vi "Finish.vi"   [LabVIEW 2019]
doc: "This VIcloses device references, sends final commands to the network tables and the joysticks, and terminates all command and control loops."
uses:
  refnums.vi
  <vilib>/Rock Robotics/WPI/Utilities/WPI_GetSetVariantRefNum.vi
types:
  T1 = typedef "WPI_ServoDeviceRef.ctl" = cluster{"DeviceStatus":errorcluster, "PWM Channel":T2, "DeadBand":T3}
  T2 = typedef "FPGA_DIOPWMChannel.ctl" = enum8{"PWM 0", "PWM 1", "PWM 2", "PWM 3", "PWM 4", "PWM 5", "PWM 6", "PWM 7", "PWM 8", "PWM 9", "PWM MXP 0", "PWM MXP 1", "PWM MXP 2", "PWM MXP 3", "PWM MXP 4", "PWM MXP 5", "PWM MXP 6", "PWM MXP 7", "PWM MXP 8", "PWM MXP 9", "Invalid"}
  T3 = typedef "WPI_PWMDeadband.ctl" = cluster{"Name":string, "maxPositivePwm":i32, "minPositivePwm":i32, "centerPwm":i32, "maxNegativePwm":i32, "minNegativePwm":i32, "angularRange":u16}
  T4 = typedef "WPI_CounterDevRef.ctl" = cluster{"DevStatus":errorcluster, "CntIndex":T5}
  T5 = typedef "FPGA_CounterCtrSystemIndex.ctl" = enum8{"Ctr 0", "Ctr 1", "Ctr 2", "Ctr 3", "Ctr 4", "Ctr 5", "Ctr 6", "Ctr 7", "Invalid"}
  T6 = typedef "WPI_SolenoidDevRef.ctl" = cluster{"DevStatus":errorcluster, "Pneumatics Control Module":u8, "Forward Solenoid Channel":T7, "Reverse Solenoid Channel":T7}
  T7 = typedef "WPI_SolenoidChannel.ctl" = enum8{"Solenoid 0", "Solenoid 1", "Solenoid 2", "Solenoid 3", "Solenoid 4", "Solenoid 5", "Solenoid 6", "Solenoid 7", "Invalid"}
  T8 = typedef "WPI_PotentiometerDevRef.ctl" = cluster{"DevStatus":errorcluster, "Analog Channel":T9, "Invert Output":bool}
  T9 = typedef "FPGA_AIChannel.ctl" = enum8{"AI 0", "AI 1", "AI 2", "AI 3", "AI MXP 0", "AI MXP 1", "AI MXP 2", "AI MXP 3", "Invalid"}
  T10 = typedef "WPI_MotorControlDeviceRef.ctl" = cluster{"DeviceStatus":errorcluster, "Type":T11, "PWM":cluster{"PWM Channel":T2, "DeadBand":T3}, "CAN":cluster{"Device Number":u8, "SetOutput VI Ref":variant, "GetOutput VI Ref":variant, "Enable VI Ref":variant, "Disable VI Ref":variant, "Data":variant}, "Invert":bool, "DIO PWM":cluster{"PWM \"Enable\" Channel":T2, "DIOChannel":T12, "PWM Rate":dbl}}
  T11 = typedef "WPI_MotorControlType.ctl" = enum16{"PWM", "CAN", "DIO PWM"}
  T12 = typedef "FPGA_DIOChannel.ctl" = enum8{"DIO 0", "DIO 1", "DIO 2", "DIO 3", "DIO 4", "DIO 5", "DIO 6", "DIO 7", "DIO 8", "DIO 9", "DIO MXP 0", "DIO MXP 1", "DIO MXP 2", "DIO MXP 3", "DIO MXP 4", "DIO MXP 5", "DIO MXP 6", "DIO MXP 7", "DIO MXP 8", "DIO MXP 9", "DIO MXP 10", "DIO MXP 11", "DIO MXP 12", "DIO MXP 13", "DIO MXP 14", "DIO MXP 15", "SPI Port CS1", "SPI Port CS2", "SPI Port CS3", "SPI Port MISO", "SPI Port MOSI", "Invalid"}
  T13 = typedef "WPI_AnalogChannelDevRef.ctl" = cluster{"DevStatus":errorcluster, "Analog Channel":T9}
  T14 = typedef "WPI_JoystickDevRef.ctl" = cluster{"Device":T15}
  T15 = typedef "WPI_JoystickDeviceEnum.ctl" = enum16{"USB 0", "USB 1", "USB 2", "USB 3", "USB 4", "USB 5"}
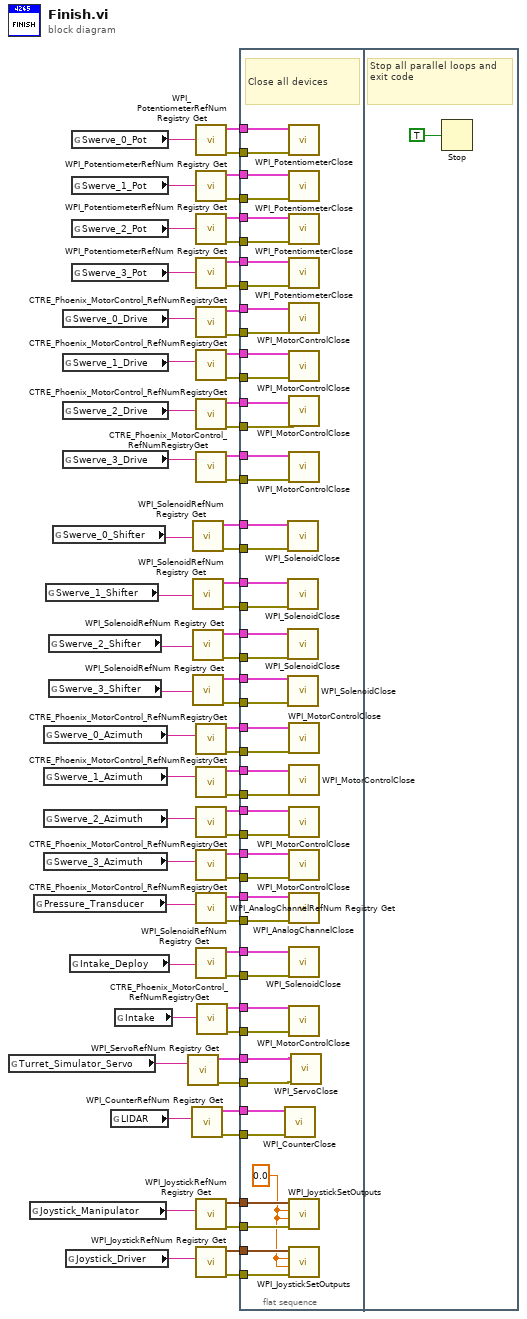
[diagram p0: block diagram]
diagram:
  n1 = global read "refnums.vi" "Turret_Simulator_Servo"() -> (w3:string)
  n2 = global read "refnums.vi" "Joystick_Manipulator"() -> (w51:string)
  n3 = global read "refnums.vi" "Pressure_Transducer"() -> (w57:string)
  n4 = global read "refnums.vi" "Swerve_0_Azimuth"() -> (w27:string)
  n5 = global read "refnums.vi" "Swerve_1_Azimuth"() -> (w26:string)
  n6 = global read "refnums.vi" "Swerve_2_Azimuth"() -> (w25:string)
  n7 = global read "refnums.vi" "Swerve_3_Azimuth"() -> (w24:string)
  n8 = global read "refnums.vi" "Swerve_1_Shifter"() -> (w11:string)
  n9 = global read "refnums.vi" "Swerve_2_Shifter"() -> (w12:string)
  n10 = global read "refnums.vi" "Swerve_3_Shifter"() -> (w39:string)
  n11 = global read "refnums.vi" "Swerve_0_Shifter"() -> (w10:string)
  n12 = global read "refnums.vi" "Swerve_0_Drive"() -> (w36:string)
  n13 = global read "refnums.vi" "Swerve_1_Drive"() -> (w33:string)
  n14 = global read "refnums.vi" "Swerve_2_Drive"() -> (w31:string)
  n15 = global read "refnums.vi" "Swerve_3_Drive"() -> (w42:string)
  n16 = global read "refnums.vi" "Joystick_Driver"() -> (w46:string)
  n17 = global read "refnums.vi" "Intake_Deploy"() -> (w54:string)
  n18 = global read "refnums.vi" "Swerve_0_Pot"() -> (w69:string)
  n19 = global read "refnums.vi" "Swerve_1_Pot"() -> (w67:string)
  n20 = global read "refnums.vi" "Swerve_2_Pot"() -> (w66:string)
  n21 = global read "refnums.vi" "Swerve_3_Pot"() -> (w65:string)
  n22 = global read "refnums.vi" "LIDAR"() -> (w45:string)
  n23 = global read "refnums.vi" "Intake"() -> (w15:string)
  n24 = call <vilib>:"WPI_ServoRefNum Registry Get.vi"("refnum name"=w3) -> ("error out"=w1:errorcluster, "ServoDeviceRef"=w2:T1)  [unwired: 9 in]
  n25 = call <vilib>:"WPI_CounterRefNum Registry Get.vi"("refnum name"=w45) -> ("error out"=w43:errorcluster, "CounterDevRef"=w44:T4)  [unwired: 9 in]
  n26 = call <vilib>:"WPI_SolenoidRefNum Registry Get.vi"("refnum name"=w10) -> ("error out"=w8:errorcluster, "SolenoidDevRef"=w9:T6)  [unwired: 9 in]
  n27 = call <vilib>:"WPI_SolenoidRefNum Registry Get.vi"("refnum name"=w11) -> ("error out"=w6:errorcluster, "SolenoidDevRef"=w7:T6)  [unwired: 9 in]
  n28 = call <vilib>:"WPI_SolenoidRefNum Registry Get.vi"("refnum name"=w12) -> ("error out"=w4:errorcluster, "SolenoidDevRef"=w5:T6)  [unwired: 9 in]
  n29 = call <vilib>:"WPI_SolenoidRefNum Registry Get.vi"("refnum name"=w39) -> ("error out"=w37:errorcluster, "SolenoidDevRef"=w38:T6)  [unwired: 9 in]
  n30 = call <vilib>:"WPI_PotentiometerRefNum Registry Get.vi"("refnum name"=w69) -> ("error out"=w61:errorcluster, "PotDevRef"=w68:T8)  [unwired: 9 in]
  n31 = call <vilib>:"WPI_PotentiometerRefNum Registry Get.vi"("refnum name"=w67) -> ("error out"=w60:errorcluster, "PotDevRef"=w64:T8)  [unwired: 9 in]
  n32 = call <vilib>:"WPI_PotentiometerRefNum Registry Get.vi"("refnum name"=w66) -> ("error out"=w59:errorcluster, "PotDevRef"=w63:T8)  [unwired: 9 in]
  n33 = call <vilib>:"WPI_PotentiometerRefNum Registry Get.vi"("refnum name"=w65) -> ("error out"=w58:errorcluster, "PotDevRef"=w62:T8)  [unwired: 9 in]
  n34 = call <vilib>:"CTRE_Phoenix_MotorControl_RefNumRegistryGet.vi"("refnum name"=w36) -> ("error out"=w34:errorcluster, "PhoenixMotorControlDevRef"=w35:T10)  [unwired: 9 in]
  n35 = call <vilib>:"CTRE_Phoenix_MotorControl_RefNumRegistryGet.vi"("refnum name"=w33) -> ("error out"=w28:errorcluster, "PhoenixMotorControlDevRef"=w32:T10)  [unwired: 9 in]
  n36 = call <vilib>:"CTRE_Phoenix_MotorControl_RefNumRegistryGet.vi"("refnum name"=w31) -> ("error out"=w29:errorcluster, "PhoenixMotorControlDevRef"=w30:T10)  [unwired: 9 in]
  n37 = call <vilib>:"CTRE_Phoenix_MotorControl_RefNumRegistryGet.vi"("refnum name"=w42) -> ("error out"=w40:errorcluster, "PhoenixMotorControlDevRef"=w41:T10)  [unwired: 9 in]
  n38 = call <vilib>:"CTRE_Phoenix_MotorControl_RefNumRegistryGet.vi"("refnum name"=w27) -> ("error out"=w19:errorcluster, "PhoenixMotorControlDevRef"=w23:T10)  [unwired: 9 in]
  n39 = call <vilib>:"CTRE_Phoenix_MotorControl_RefNumRegistryGet.vi"("refnum name"=w26) -> ("error out"=w18:errorcluster, "PhoenixMotorControlDevRef"=w22:T10)  [unwired: 9 in]
  n40 = call <vilib>:"CTRE_Phoenix_MotorControl_RefNumRegistryGet.vi"("refnum name"=w25) -> ("error out"=w17:errorcluster, "PhoenixMotorControlDevRef"=w21:T10)  [unwired: 9 in]
  n41 = call <vilib>:"CTRE_Phoenix_MotorControl_RefNumRegistryGet.vi"("refnum name"=w24) -> ("error out"=w16:errorcluster, "PhoenixMotorControlDevRef"=w20:T10)  [unwired: 9 in]
  n42 = call <vilib>:"WPI_AnalogChannelRefNum Registry Get.vi"("refnum name"=w57) -> ("error out"=w55:errorcluster, "AIDeviceRef"=w56:T13)  [unwired: 9 in]
  n43 = call <vilib>:"WPI_SolenoidRefNum Registry Get.vi"("refnum name"=w54) -> ("error out"=w52:errorcluster, "SolenoidDevRef"=w53:T6)  [unwired: 9 in]
  n44 = call <vilib>:"WPI_JoystickRefNum Registry Get.vi"("refnum name"=w51) -> ("error out"=w49:errorcluster, "JoystickDevRef"=w50:T14)  [unwired: 9 in]
  n45 = call <vilib>:"WPI_JoystickRefNum Registry Get.vi"("refnum name"=w46) -> ("error out"=w47:errorcluster, "JoystickDevRef"=w48:T14)  [unwired: 9 in]
  n46 = call <vilib>:"CTRE_Phoenix_MotorControl_RefNumRegistryGet.vi"("refnum name"=w15) -> ("error out"=w13:errorcluster, "PhoenixMotorControlDevRef"=w14:T10)  [unwired: 9 in]
  n47 = flat-sequence {
    tunnel: w68 -> [w116]
    tunnel: w64 -> [w115]
    tunnel: w63 -> [w114]
    tunnel: w62 -> [w113]
    tunnel: w35 -> [w112]
    tunnel: w32 -> [w111]
    tunnel: w61 -> [w110]
    tunnel: w60 -> [w109]
    tunnel: w59 -> [w108]
    tunnel: w58 -> [w107]
    tunnel: w34 -> [w106]
    tunnel: w56 -> [w105]
    tunnel: w55 -> [w104]
    tunnel: w53 -> [w103]
    tunnel: w52 -> [w102]
    tunnel: w50 -> [w101]
    tunnel: w49 -> [w100]
    tunnel: w48 -> [w99]
    tunnel: w47 -> [w98]
    tunnel: w44 -> [w96]
    tunnel: w43 -> [w95]
    tunnel: w41 -> [w94]
    tunnel: w40 -> [w93]
    tunnel: w38 -> [w92]
    tunnel: w37 -> [w91]
    tunnel: w30 -> [w90]
    tunnel: w29 -> [w89]
    tunnel: w28 -> [w88]
    tunnel: w23 -> [w87]
    tunnel: w22 -> [w86]
    tunnel: w21 -> [w85]
    tunnel: w20 -> [w84]
    tunnel: w19 -> [w83]
    tunnel: w18 -> [w82]
    tunnel: w17 -> [w81]
    tunnel: w16 -> [w80]
    tunnel: w14 -> [w79]
    tunnel: w13 -> [w78]
    tunnel: w9 -> [w77]
    tunnel: w8 -> [w76]
    tunnel: w7 -> [w75]
    tunnel: w6 -> [w74]
    tunnel: w5 -> [w73]
    tunnel: w4 -> [w72]
    tunnel: w2 -> [w71]
    tunnel: w1 -> [w70]
    frame #0 {
      w97 = sgl 0.0 ("Left Rumble")
      # "Close all devices"
      n48 = call <vilib>:"WPI_CounterClose.vi"("error in (no error)"=w95, "CounterDevRef"=w96) -> ()  [unwired: 9 in, 1 out]
      n49 = call <vilib>:"WPI_SolenoidClose.vi"("error in (no error)"=w76, "SolenoidDevRef"=w77) -> ()  [unwired: 9 in, 1 out]
      n50 = call <vilib>:"WPI_SolenoidClose.vi"("error in (no error)"=w74, "SolenoidDevRef"=w75) -> ()  [unwired: 9 in, 1 out]
      n51 = call <vilib>:"WPI_SolenoidClose.vi"("error in (no error)"=w72, "SolenoidDevRef"=w73) -> ()  [unwired: 9 in, 1 out]
      n52 = call <vilib>:"WPI_SolenoidClose.vi"("error in (no error)"=w91, "SolenoidDevRef"=w92) -> ()  [unwired: 9 in, 1 out]
      n53 = call <vilib>:"WPI_PotentiometerClose.vi"("error in"=w110, "PotDevRef"=w116) -> ()  [unwired: 9 in, 1 out]
      n54 = call <vilib>:"WPI_PotentiometerClose.vi"("error in"=w109, "PotDevRef"=w115) -> ()  [unwired: 9 in, 1 out]
      n55 = call <vilib>:"WPI_PotentiometerClose.vi"("error in"=w108, "PotDevRef"=w114) -> ()  [unwired: 9 in, 1 out]
      n56 = call <vilib>:"WPI_PotentiometerClose.vi"("error in"=w107, "PotDevRef"=w113) -> ()  [unwired: 9 in, 1 out]
      n57 = call <vilib>:"WPI_MotorControlClose.vi"("error in"=w106, "MotorControlDevRef"=w112) -> ()  [unwired: 9 in, 1 out]
      n58 = call <vilib>:"WPI_MotorControlClose.vi"("error in"=w88, "MotorControlDevRef"=w111) -> ()  [unwired: 9 in, 1 out]
      n59 = call <vilib>:"WPI_MotorControlClose.vi"("error in"=w89, "MotorControlDevRef"=w90) -> ()  [unwired: 9 in, 1 out]
      n60 = call <vilib>:"WPI_MotorControlClose.vi"("error in"=w93, "MotorControlDevRef"=w94) -> ()  [unwired: 9 in, 1 out]
      n61 = call <vilib>:"WPI_MotorControlClose.vi"("error in"=w83, "MotorControlDevRef"=w87) -> ()  [unwired: 9 in, 1 out]
      n62 = call <vilib>:"WPI_MotorControlClose.vi"("error in"=w82, "MotorControlDevRef"=w86) -> ()  [unwired: 9 in, 1 out]
      n63 = call <vilib>:"WPI_MotorControlClose.vi"("error in"=w81, "MotorControlDevRef"=w85) -> ()  [unwired: 9 in, 1 out]
      n64 = call <vilib>:"WPI_MotorControlClose.vi"("error in"=w80, "MotorControlDevRef"=w84) -> ()  [unwired: 9 in, 1 out]
      n65 = call <vilib>:"WPI_AnalogChannelClose.vi"("error in (no error)"=w104, "AIDeviceRef"=w105) -> ()  [unwired: 9 in, 1 out]
      n66 = call <vilib>:"WPI_SolenoidClose.vi"("error in (no error)"=w102, "SolenoidDevRef"=w103) -> ()  [unwired: 9 in, 1 out]
      n67 = call <vilib>:"WPI_MotorControlClose.vi"("error in"=w78, "MotorControlDevRef"=w79) -> ()  [unwired: 9 in, 1 out]
      n68 = call <vilib>:"WPI_JoystickSetOutputs.vi"("error in (no error)"=w100, "Right Rumble"=w97, "Left Rumble"=w97, "JoystickDevRef"=w101) -> ()  [unwired: 6 in, 2 out]
      n69 = call <vilib>:"WPI_JoystickSetOutputs.vi"("error in (no error)"=w98, "Right Rumble"=w97, "Left Rumble"=w97, "JoystickDevRef"=w99) -> ()  [unwired: 6 in, 2 out]
      n70 = call <vilib>:"WPI_ServoClose.vi"("error in (no error)"=w70, "ServoDeviceRef"=w71) -> ()  [unwired: 9 in, 1 out]
    }
    frame #1 {
      # "Stop all parallel loops and exit code"
      n71 = Stop(stop? (T)=TRUE ("Quit")) -> ()
    }
  }
